vi "get_scan_duration.vi"(8 "error in (no error)":errorcluster, 11 "GenericTrajectory in":refnum<class "GenericTrajectory.lvclass">) -> (0 "error out":errorcluster, 2 "scan duration":dbl[unit], 3 "GenericTrajectory out":refnum<class "GenericTrajectory.lvclass">)   [LabVIEW 2010, in "GenericTrajectory.lvclass"]
doc: "returns the duration of a single scan performed in one piece when in single-sweep mode or experiment mode"
uses:
  GenericTrajectory.lvclass
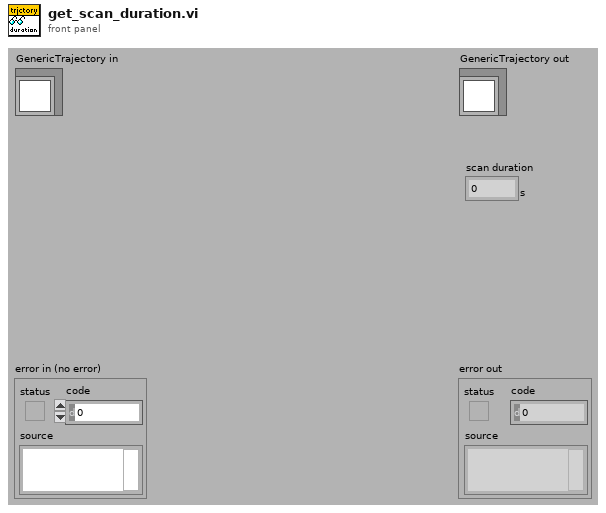
[diagram p1: front panel]
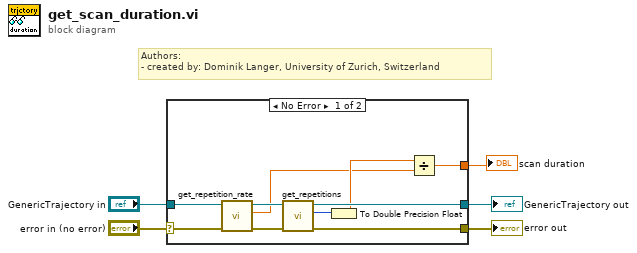
[diagram p0: block diagram]
diagram:
  # "Authors: \n- created by: Dominik Langer, University of Zurich, Switzerland"
  n1 = case shown="No Error" "error in (no error)" {
    selector: "error in (no error)" -> [w11 w17]
    tunnel: [w10 w17] -> w4
    tunnel: [w13 w16] -> w2
    tunnel: "GenericTrajectory in" -> [w14 w16]
    tunnel: [w6 _] -> w1
    frame No Error {
      n2 = call-dynamic "get_repetition_rate.vi"("error in (no error)"=w11, "GenericTrajectory in"=w14) -> ("error out"=w12:errorcluster, "repetition rate"=w7:dbl[unit], "GenericTrajectory out"=w15:refnum<class "GenericTrajectory.lvclass">)  [unwired: 7 in]
      n3 = call-dynamic "get_repetitions.vi"("error in (no error)"=w12, "GenericTrajectory in"=w15) -> ("error out"=w10:errorcluster, "repetitions"=w9:i32, "GenericTrajectory out"=w13:refnum<class "GenericTrajectory.lvclass">)  [unwired: 7 in]
      n4 = To Double Precision Float(number=w9) -> (double precision float=w8:dbl)
      n5 = Divide(x=w8, y=w7) -> (x/y=w6:dbl[unit])
    }
    frame Error {
    }
  }
  "error out" <- w4
  "GenericTrajectory out" <- w2
  "scan duration" <- w1
